vi "Solve1.vi"(8 "Error In":errorcluster, 11 "object in":refnum<class "2024_19.lvclass">) -> (0 "Error Out":errorcluster, 2 "Result":u64, 3 "object out":refnum<class "2024_19.lvclass">)   [LabVIEW 2023, in "2024_19.lvclass"]
uses:
  2024_19.lvclass
  2024_19.lvclass/2024_19.ctl
panel:
  out "Numeric":i32
  out "Makable":bool
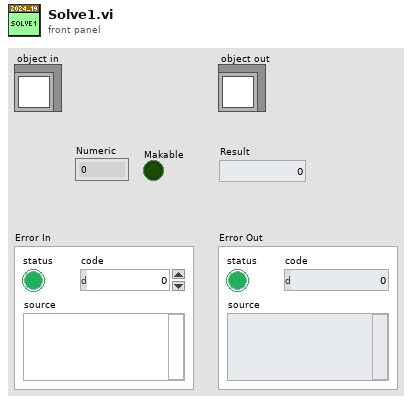
[diagram p1: front panel]
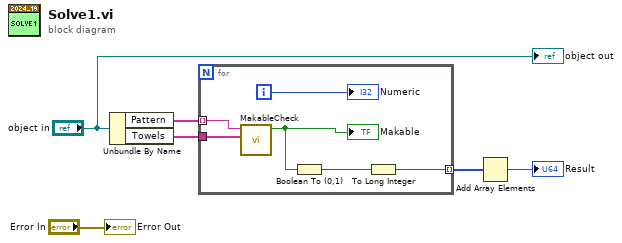
[diagram p0: block diagram]
diagram:
  n1 = Unbundle By Name("object in") -> ("Pattern"=w2:string[], "Towels"=w1:string[])
  n2 = for {
    tunnel: w1 -> [w12]
    tunnel: w2 -> [w11] mode=indexing
    tunnel: [w7] -> w4 mode=indexing
    i -> [w10]
    n3 = call "MakableCheck.vi"("Towels"=w12, "Pattern"=w11) -> ("Makable"=w9:bool)  [unwired: 9 in]
    "Makable" <- w9
    n4 = Boolean To (0,1)(Boolean=w9) -> (0, 1=w8:i16)
    n5 = To Long Integer(number=w8) -> (32bit integer=w7:i32)
    "Numeric" <- w10
  }
  n6 = Add Array Elements(numeric array=w4) -> (sum=→"Result":i32)
  "Error Out" <- "Error In"
  "object out" <- "object in"
